vi "Stop Sweep Waveform.vi"(8 "error in (no error)":errorcluster, 10 "Waveforms in":waveform(dbl)[](array[waveform]), 11 "Instrument.DAQ in":refnum<class "Instrument.DAQ.lvclass">) -> (0 "error out":errorcluster, 2 "Waveforms out":waveform(dbl)[](array[waveform]), 3 "Instrument.DAQ out":refnum<class "Instrument.DAQ.lvclass">)   [LabVIEW 2019, in "Instrument.Lockin.lvlib" / "Instrument.DAQ.lvclass"]
uses:
  Instrument.DAQ.lvclass
  Instrument.DAQ.lvclass/Instrument.DAQ.ctl
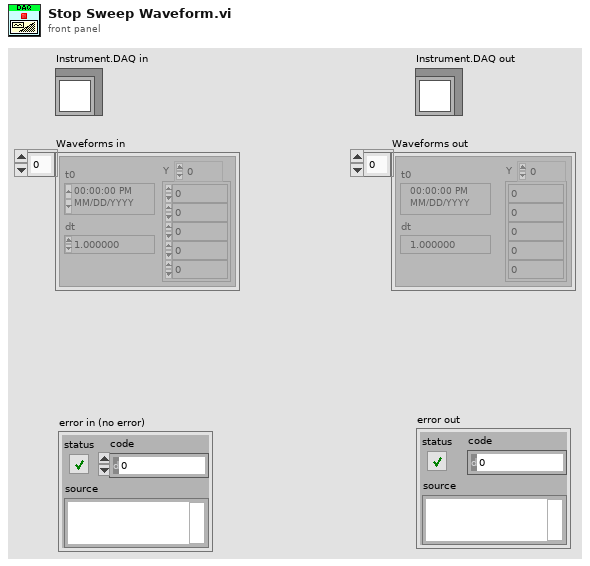
[diagram p1: front panel]
types:
  T1 = typedef "Instrument.Lockin.lvlib/Instrument.DAQ.lvclass/Sweep.Channel--Cluster--Array.ctl" = T2[]
  T2 = typedef "Instrument.Lockin.lvlib/Instrument.DAQ.lvclass/Sweep.Channel--Cluster.ctl" = cluster{"Enable?":bool, "Channel":u16, "Start":dbl, "End":dbl, "Pattern":T3, "Table":dbl[]}
  T3 = typedef "Instrument.Lockin.lvlib/Instrument.DAQ.lvclass/Sweep.Pattern--Enum.ctl" = enum16{"Ramp /", "Ramp /\\", "Smooth Ramp _/", "Smooth Ramp _/\\_", "Table"}
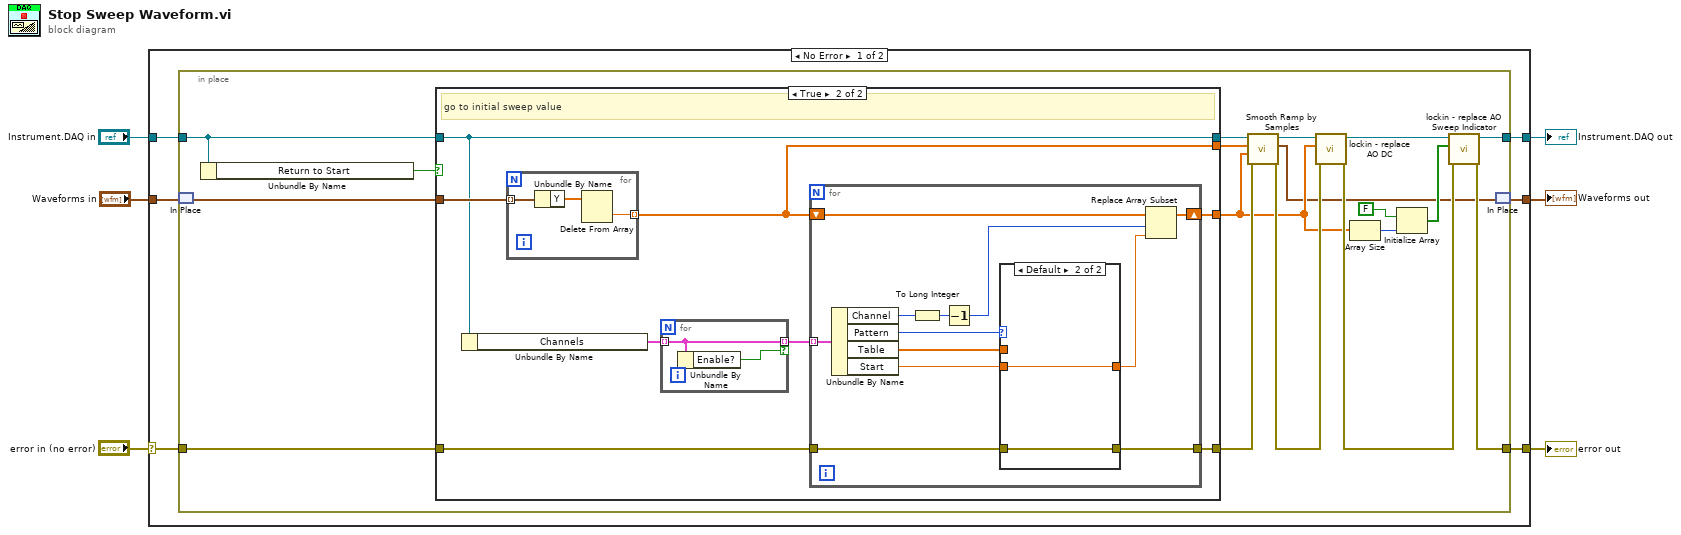
[diagram p0: block diagram]
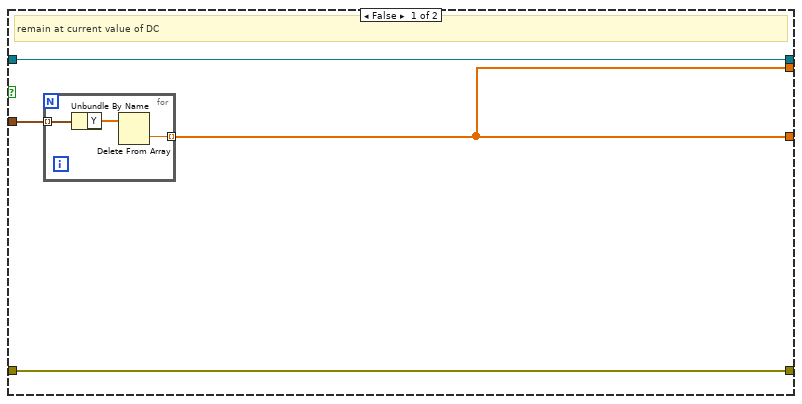
[diagram p2: hidden frame]
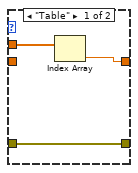
[diagram p3: hidden frame]
diagram:
  n1 = case shown="No Error" "error in (no error)" {
    selector: "error in (no error)" -> [w12 w69]
    tunnel: "Instrument.DAQ in" -> [w11 w68]
    tunnel: [w10 w68] -> w4
    tunnel: [w7 _] -> w3
    tunnel: [w9 w69] -> w2
    tunnel: "Waveforms in" -> [w8 _]
    frame No Error {
      n2 = in-place {
        in-place-border: w12 -> [w30]
        in-place-border: w11 -> [w28]
        in-place-border: [w27] -> w10
        in-place-border: [w26] -> w9
        n3 = in-place-match #1(w8) -> (w14:waveform(dbl)[])
        n4 = Unbundle By Name(w28) -> ("Return to Start"=w29:bool)
        n5 = case shown="True" w29 {
          tunnel: w30 -> [w33 w45]
          tunnel: [w33 w41] -> w22
          tunnel: w28 -> [w34 w40]
          tunnel: [w34 w40] -> w24
          tunnel: w14 -> [w32 w42]
          tunnel: [w31 w39] -> w21
          tunnel: [w31 w38] -> w15
          frame False {
            # "remain at current value of DC"
            n6 = for {
              tunnel: w32 -> [w37] mode=indexing
              tunnel: [w35] -> w31 mode=indexing
              n7 = Unbundle By Name(w37) -> ("Y"=w36:dbl[])
              n8 = Delete From Array(array=w36) -> (deleted portion=w35:dbl)  [unwired: 2 in, 1 out]
            }
          }
          frame True {
            # "go to initial sweep value"
            n9 = Unbundle By Name(w40) -> ("Channels"=w44:T1)
            n10 = for {
              tunnel: w42 -> [w48] mode=indexing
              tunnel: [w46] -> w39 mode=indexing
              n11 = Unbundle By Name(w48) -> ("Y"=w47:dbl[])
              n12 = Delete From Array(array=w47) -> (deleted portion=w46:dbl)  [unwired: 2 in, 1 out]
            }
            n13 = for {
              tunnel: w44 -> [w67] mode=indexing
              tunnel: [w67] -> w43 mode=indexing if=w66
              n14 = Unbundle By Name(w67) -> ("Enable?"=w66:bool)
            }
            n15 = for {
              tunnel: w43 -> [w57] mode=indexing
              tunnel: w45 -> [w60]
              tunnel: [w56] -> w41
              shift-right: [w50] -> w38
              shift-left: w39 -> [w49]
              n16 = Unbundle By Name(w57) -> ("Channel"=w58:u16, "Pattern"=w55:T3, "Table"=w54:dbl[], "Start"=w53:dbl)
              n17 = To Long Integer(number=w58) -> (32bit integer=w59:i32)
              n18 = Decrement(x=w59) -> (x-1=w52:i32)
              n19 = case shown="Default" w55 {
                tunnel: [w61 w64] -> w56
                tunnel: w60 -> [w61 w64]
                tunnel: w54 -> [w63 _]
                tunnel: w53 -> [_ w65]
                tunnel: [w62 w65] -> w51
                frame "Table" {
                  n20 = Index Array(array=w63) -> (element=w62:dbl)  [unwired: 1 in]
                }
                frame Default {
                }
              }
              n21 = Replace Array Subset(array=w49, new element=w51, index=w52) -> (w50:dbl[])
            }
          }
        }
        n22 = call "Smooth Ramp by Samples.vi"("error in (no error)"=w22, "End"=w15, "Start"=w21, "Instrument.DAQ"=w24) -> ("Error out"=w23:errorcluster, "Waveforms out"=w13:waveform(dbl)[], "Instrument.DAQ out"=w25:refnum<class "Instrument.DAQ.lvclass">)  [unwired: 5 in]
        n23 = call "lockin - replace AO DC.vi"("error in (no error)"=w23, "AO.DC (V)"=w15, "Instrument.DAQ"=w25) -> ("error out"=w16:errorcluster, "Instrument.DAQ out"=w18:refnum<class "Instrument.DAQ.lvclass">)  [unwired: 7 in]
        n24 = Array Size(array=w15) -> (size(s)=w19:i32)
        n25 = Initialize Array(FALSE, w19) -> (w17:bool[])
        n26 = call "lockin - replace AO Sweep Indicator.vi"("error in (no error)"=w16, "Channels: AO.Sweeping?"=w17, "Instrument.DAQ"=w18) -> ("error out"=w26:errorcluster, "Instrument.DAQout"=w27:refnum<class "Instrument.DAQ.lvclass">)  [unwired: 7 in]
        n27 = in-place-match #1(w13) -> (w7:waveform(dbl)[])
      }
    }
    frame Error {
    }
  }
  "error out" <- w2
  "Instrument.DAQ out" <- w4
  "Waveforms out" <- w3
